vi "Set Home.vi"() -> ()   [LabVIEW 2017, in "Stage.lvlib"]
uses:
  Stage.lvlib
  Drivers/ASI/ASI TG-1000.lvlib
panel:
  out "VISA out":refnum<visa-resource-name>
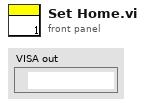
[diagram p1: front panel]
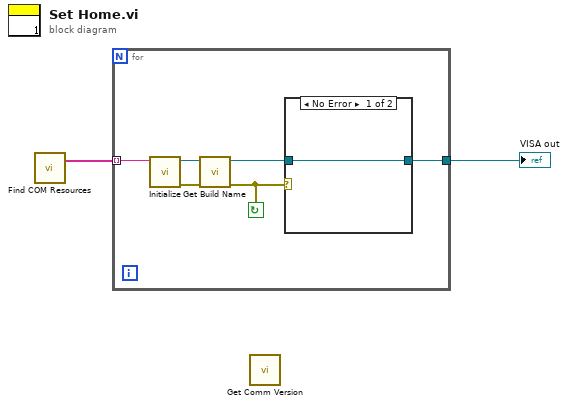
[diagram p0: block diagram]
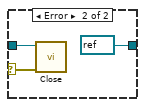
[diagram p2: hidden frame]
diagram:
  n1 = call "Find COM Resources.vi"() -> ("COM only list"=w2:string[])  [unwired: 2 in, 1 out]
  n2 = for {
    tunnel: w2 -> [w8] mode=indexing
    tunnel: [w5] -> w1
    stop <- w3 continue-if-true
    n3 = call "Initialize.vi"("VISA resource name"=w8) -> ("error out"=w6:errorcluster, "VISA resource name out"=w7:refnum<visa-resource-name>)  [unwired: 9 in]
    n4 = call "Get Build Name.vi"("error in (no error)"=w6, "VISA in"=w7) -> ("error out"=w3:errorcluster, "VISA out"=w4:refnum<visa-resource-name>)  [unwired: 6 in, 1 out]
    n5 = case shown="No Error" w3 {
      selector: w3 -> [_ w12]
      tunnel: [w9 refnum<visa-resource-name> refnum ("VISA out")] -> w5
      tunnel: w4 -> [w9 w11]
      frame No Error {
      }
      frame Error {
        n6 = call "Close.vi"("error in (no error)"=w12, "VISA resource name"=w11) -> ()  [unwired: 9 in, 1 out]
      }
    }
  }
  "VISA out" <- w1
  n7 = call "Get Comm Version.vi"() -> ()  [unwired: 8 in, 3 out]
